vi "Obtain Execution Notifier.vi"() -> (3 "Execution Notifier":refnum<notifier>)   [LabVIEW 2017, in "LVUnit Test Executor.Tests.lvlib"]
uses:
  LVUnit Test Executor.Tests.lvlib
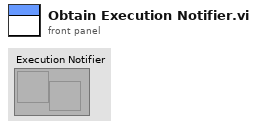
[diagram p1: front panel]
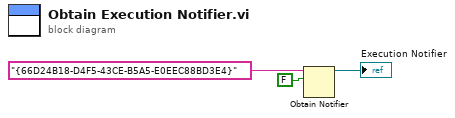
[diagram p0: block diagram]
diagram:
  n1 = Obtain Notifier(name (unnamed)="{66D24B18-D4F5-43CE-B5A5-E0EEC88BD3E4}", notification data type=FALSE) -> (notifier out=→"Execution Notifier":refnum<notifier>)  [unwired: 2 in, 2 out]
